vi "Read Samples (Complex DBL Waveform).vi"(8 "error in (no error)":errorcluster, 10 "Samples":i32, 11 "RTL-SDR in":refnum<class "Session.lvclass">) -> (0 "error out":errorcluster, 2 "Complex DBL Waveform":cluster{"x0":dbl, "dx":dbl, "[y]":cdb[]}, 3 "RTL-SDR out":refnum<class "Session.lvclass">)   [LabVIEW 2020, in "RTL-SDR.lvlib" / "Session.lvclass"]
uses:
  Session.lvclass
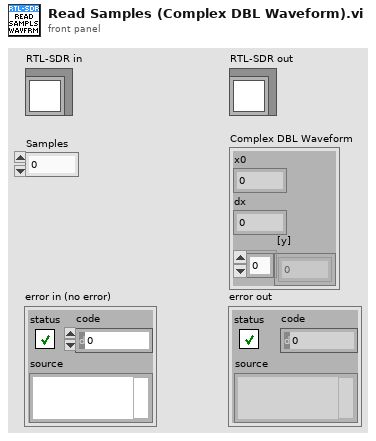
[diagram p1: front panel]
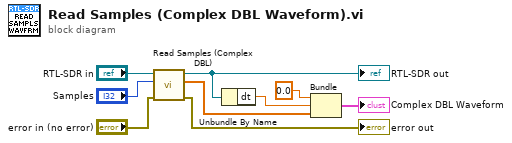
[diagram p0: block diagram]
diagram:
  n1 = call "Read Samples (Complex DBL).vi"("error in (no error)"="error in (no error)", "Samples"="Samples", "RTL-SDR in"="RTL-SDR in") -> ("error out"=→"error out":errorcluster, "Complex Array"=w4:cdb[], "RTL-SDR out"=w2:refnum<class "Session.lvclass">)  [unwired: 6 in]
  "RTL-SDR out" <- w2
  n2 = Unbundle By Name(w2) -> ("dt"=w5:dbl)
  n3 = Bundle(0.0, "dt"=w5, "Complex Array"=w4) -> (→"Complex DBL Waveform":cluster{dbl, "dt":dbl, "Complex Array":cdb[]})  [unwired: 1 in]
